vi "Thev-Next Step.vi"(0 "State in":T1, 5 "Params":T5 {"LProbe" items=["None"=-1, "Probe A"=0, "Probe B"=1]; "Rprobe" items=["None"=-1, "Probe A"=0, "Probe B"=1]}) -> (4 "State out":T1, 6 "Navgs":i32, 8 "Path":path, 15 "error out":errorcluster)   [LabVIEW 2015]
uses:
  Typedefs/Thev-Parameters.ctl
  Typedefs/Thev-Stimulus.ctl
  Typedefs/Thev-Find.ctl
  Misc VIs/Equipment Control/ER10X/ER10X-Probe.ctl
  Typedefs/Thev-Optimization Parameters.ctl
  Typedefs/Thev-State.ctl
  D:/Experiment VIs/Misc VIs/Equipment Control/ER10X/ER10XConnect.NET.dll
  Misc VIs/Equipment Control/ER10X/ER10XConnect.NET.dll
  Typedefs/Thev-Procedure Phase.ctl
  Typedefs/Thev-Progress Table Element.ctl
  Typedefs/Thev-Optimization Result.ctl
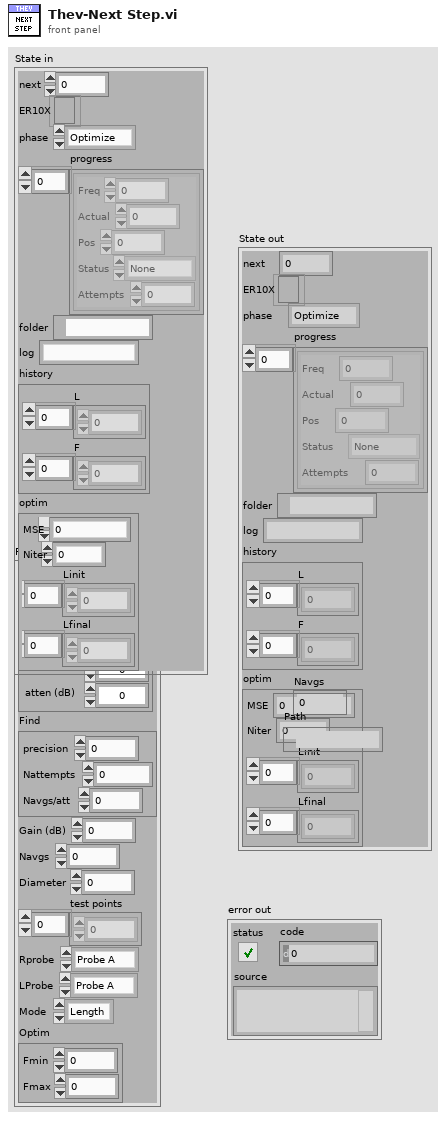
[diagram p1: front panel]
types:
  T1 = typedef "Thev-State.ctl" = cluster{"next":i32, "ER10X":refnum<k24>, "phase":T2, "progress":T3[], "folder":path, "log":string, "history":cluster{"L":dbl[], "F":dbl[]}, "optim":T4}
  T2 = typedef "Thev-Procedure Phase.ctl" = enum16{"Optimize", "Measure", "Compute", "Finished"}
  T3 = typedef "Thev-Progress Table Element.ctl" = cluster{"Freq":dbl, "Actual":dbl, "Pos":dbl, "Status":enum16{"None", "Measuring", "Finished"}, "Attempts":i32}
  T4 = typedef "Thev-Optimization Result.ctl" = cluster{"MSE":dbl, "Niter":i32, "Linit":dbl[], "Lfinal":dbl[]}
  T5 = typedef "Thev-Parameters.ctl" = cluster{"Speaker":enum16{"Right primary", "Right secondary", "Left primary", "Left secondary"}, "Chirp":T6, "Find":T7, "Gain (dB)":dbl, "Navgs":i32, "Diameter":dbl, "test points":dbl[], "Rprobe":T8, "LProbe":T8, "Mode":enum16{"Length", "Freq"}, "Optim":T9}
  T6 = typedef "Thev-Stimulus.ctl" = cluster{"resol (Hz)":dbl, "atten (dB)":dbl, "Fs (Hz)":dbl}
  T7 = typedef "Thev-Find.ctl" = cluster{"precision":dbl, "Nattempts":i32, "Navgs/att":i32}
  T8 = typedef "ER10X-Probe.ctl" = i32
  T9 = typedef "Thev-Optimization Parameters.ctl" = cluster{"Fmin":dbl, "Fmax":dbl}
  T10 = enum16{"Right primary", "Right secondary", "Left primary", "Left secondary"}
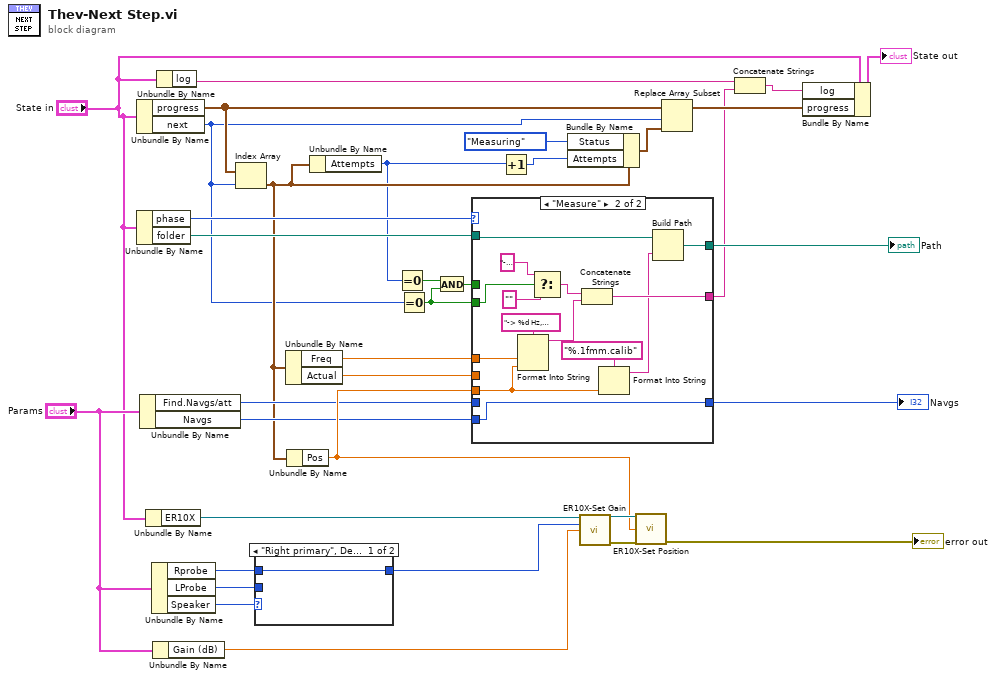
[diagram p0: block diagram]
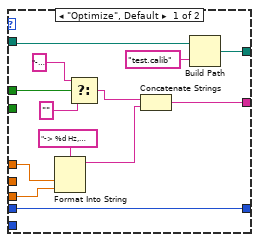
[diagram p2: hidden frame]
diagram:
  n1 = Unbundle By Name("State in") -> ("progress"=w24:T3[], "next"=w5:i32)
  n2 = Unbundle By Name("State in") -> ("phase"=w20:T2, "folder"=w19:path)
  n3 = Unbundle By Name("Params") -> ("Find.Navgs/att"=w14:i32, "Navgs"=w15:i32)
  n4 = Unbundle By Name("State in") -> ("ER10X"=w32:refnum<k24>)
  n5 = Unbundle By Name("Params") -> ("Rprobe"=w33:T8, "LProbe"=w34:T8, "Speaker"=w35:T10)
  n6 = Unbundle By Name("Params") -> ("Gain (dB)"=w30:dbl)
  n7 = Unbundle By Name("State in") -> ("log"=w11:string)
  n8 = Index Array(array=w24, index=w5) -> (element=w8:T3)
  n9 = case shown="\"Right primary\", Default" w35 {
    tunnel: w34 -> [_ w37]
    tunnel: w33 -> [w36 _]
    tunnel: [w36 w37] -> w31
    frame "Right primary", Default {
    }
    frame "Left primary", "Left secondary" {
    }
  }
  n10 = Unbundle By Name(w8) -> ("Freq"=w16:dbl, "Actual"=w2:dbl)
  n11 = Unbundle By Name(w8) -> ("Pos"=w17:dbl)
  n12 = Unbundle By Name(w8) -> ("Attempts"=w6:i32)
  n13 = Equal To 0?(x=w6) -> (x = 0?=w4:bool)
  n14 = Equal To 0?(x=w5) -> (x = 0?=w1:bool)
  n15 = And(x=w4, y=w1) -> (x .and. y?=w3:bool)
  n16 = case shown="\"Measure\"" w20 {
    tunnel: w19 -> [w50 w64]
    tunnel: [w48 w63] -> w18
    tunnel: w17 -> [w45 w53]
    tunnel: w16 -> [w46 w61]
    tunnel: [w40 w56] -> w10
    tunnel: w15 -> [_ w55]
    tunnel: w14 -> [w39 _]
    tunnel: [w39 w55] -> w13
    tunnel: w3 -> [w38 _]
    tunnel: w2 -> [_ _]
    tunnel: w1 -> [_ w51]
    frame "Optimize", Default {
      n17 = Format Into String(format string="-> %d Hz, %.1f mm", w46, w45) -> (resulting string=w41:string)  [unwired: 2 in, 1 out]
      n18 = Select(t="---Optimize lengths---\n", s=w38, f="") -> (s? t:f=w42:string)
      n19 = Concatenate Strings(w42, w41) -> (w40:string)
      n20 = Build Path(base path=w50, name or relative path="test.calib") -> (appended path=w48:path)
    }
    frame "Measure" {
      n21 = Format Into String(format string="-> %d Hz, %.1f mm", w61, w53) -> (resulting string=w57:string)  [unwired: 2 in, 1 out]
      n22 = Select(t="---Measure final---\n", s=w51, f="") -> (s? t:f=w58:string)
      n23 = Concatenate Strings(w58, w57) -> (w56:string)
      n24 = Format Into String(format string="%.1fmm.calib", w53) -> (resulting string=w52:string)  [unwired: 2 in, 1 out]
      n25 = Build Path(base path=w64, name or relative path=w52) -> (appended path=w63:path)
    }
  }
  "Navgs" <- w13
  "Path" <- w18
  n26 = Increment(x=w6) -> (x+1=w7:i32)
  n27 = Bundle By Name(cluster=w8, "Status"=enum16{"None", "Measuring", "Finished"}."Measuring", "Attempts"=w7) -> (w23:T3)
  n28 = call "ER10X-Set Gain.vi"("ER10X"=w32, "probe"=w31, "gain"=w30) -> ("reference out"=w29:refnum<k24>, "error out"=w28:errorcluster)  [unwired: 11 in]
  n29 = call "ER10X-Set Position.vi"("ER10X"=w29, "length"=w17, "error in (no error)"=w28) -> ("error out"=→"error out":errorcluster)  [unwired: 11 in, 1 out]
  n30 = Replace Array Subset(array=w24, new element=w23, index=w5) -> (w21:T3[])
  n31 = Concatenate Strings(w11, w10) -> (w9:string)
  n32 = Bundle By Name(cluster="State in", "log"=w9, "progress"=w21) -> (→"State out":T1)
